vi "__DataToVAttrbutes.vi"(8 "error in (no error)":errorcluster, 11 "data":variant) -> (0 "error out":errorcluster, 3 "VAttributes":variant)   [LabVIEW 2019, in "lv-apt-json-file.lvlib"]
uses:
  lv-apt-json-file.lvlib
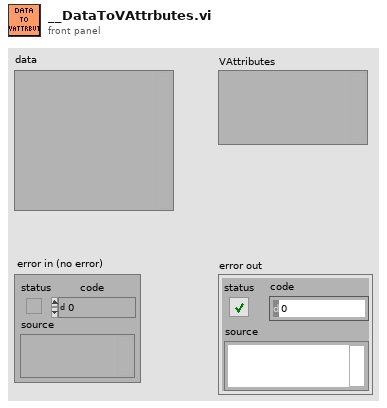
[diagram p1: front panel]
types:
  T1 = typedef "Type Descriptor Enumeration__ogtk.ctl" = enum8{"<Null>", "I8", "I16", "I32", "I64", "U8", "U16", "U32", "U64", "SGL", "DBL", "EXT", "CSG", "CDB", "CXT", "0x0F", "0x10", "0x11", "0x12", "0x13", "0x14", "Enum U8", "Enum U16", "Enum U32", "Enum U64", "SGL PQ", "DBL PQ", "EXT PQ", "CSG PQ", "CDB PQ", "CXT PQ", "0x1F", "0x20", "Boolean", "0x22", "0x23", "0x24", "0x25", "0x26", "0x27", "0x28", "0x29", "0x2A", "0x2B", "0x2C", "0x2D", "0x2E", "0x2F", "String", "0x31", "Path", "Pict", "0x34", "0x35", "0x36", "DAQ", "0x38", "0x39", "0x3A", "0x3B", "0x3C", "0x3D", "0x3E", "0x3F", "Array", "0x41", "0x42", "0x43", "0x44", "0x45", "0x46", "0x47", "0x48", "0x49", "0x4A", "0x4B", "0x4C", "0x4D", "0x4E", "0x4F", "Cluster", "0x51", "0x52", "Variant", "Waveform", "0x55", "0x56", "0x57", "0x58", "0x59", "0x5A", "0x5B", "0x5C", "0x5D", "0x5E", "0x5F", "0x60", "0x61", "0x62", "0x63", "0x64", "0x65", "0x66", "0x67", "0x68", "0x69", "0x6A", "0x6B", "0x6C", "0x6D", "0x6E", "0x6F", "Refnum"}
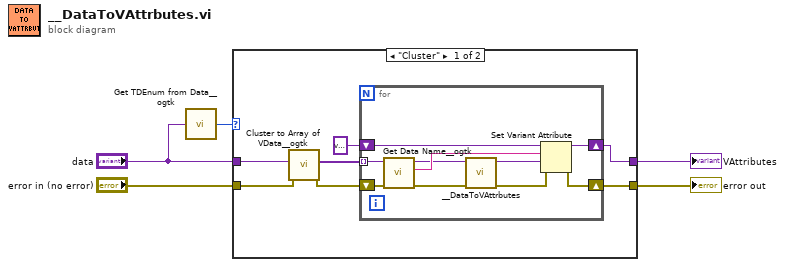
[diagram p0: block diagram]
diagram:
  n1 = call <userlib>:"Get TDEnum from Data__ogtk.vi"("Data"="data") -> ("Type Descriptor Enumeration"=w5:T1)  [unwired: 4 in]
  n2 = case shown="\"Cluster\"" w5 {
    tunnel: "data" -> [w12 w24]
    tunnel: [w9 w24] -> w3
    tunnel: [w6 w23] -> w2
    tunnel: "error in (no error)" -> [w8 w23]
    frame "Cluster" {
      n3 = call <userlib>:"Cluster to Array of VData__ogtk.vi"("error in (no error)"=w8, "Cluster"=w12) -> ("error out"=w7:errorcluster, "Array of VData"=w11:variant[])  [unwired: 8 in]
      n4 = for {
        tunnel: w11 -> [w22] mode=indexing
        shift-right: [w19] -> w9
        shift-left: variant ("variant") -> [w20]
        shift-right: [w13] -> w6
        shift-left: w7 -> [w14]
        n5 = call <userlib>:"Get Data Name__ogtk.vi"("error in (no error)"=w14, "Data"=w22) -> ("error out"=w15:errorcluster, "Data Name"=w21:string, "Data dup"=w18:variant)  [unwired: 7 in]
        n6 = call "__DataToVAttrbutes.vi"("error in (no error)"=w15, "data"=w18) -> ("error out"=w16:errorcluster, "VAttributes"=w17:variant)  [unwired: 8 in]
        n7 = Set Variant Attribute(Variant=w20, name=w21, value=w17, error in=w16) -> (Variant out=w19:variant, error out=w13:errorcluster)  [unwired: 1 out]
      }
    }
    frame Default {
    }
  }
  "VAttributes" <- w3
  "error out" <- w2
